vi "FINAL.vi"() -> ()   [LabVIEW 2011]
uses:
  <vilib>/Instr/_visa.llb/VISA Configure Serial Port (Instr).vi
panel:
  out "Light Sensor":dbl(slide) scale=0.0..1500.0
  out "Pressure":dbl(knob) scale=0.0..150000.0
  in  "flow control":u16(ring) items=["None"=0, "XON/XOFF"=1, "RTS/CTS"=2, "DTR/DSR"=4]
  in  "stop bits":u16(ring)=10 items=["1.0"=10, "1.5"=15, "2.0"=20]
  in  "parity":u16(ring) items=["None", "Odd", "Even", "Mark", "Space"]
  in  "data bits":u16=8 min=5 max=8 step=1
  in  "read":bool=TRUE
  out "bytes read":u32
  out "read string":string
  in  "VISA resource name":refnum<visa-resource-name>="COM1"
  in  "baud rate":u32=9600
  out "?":dbl
  out "?":dbl
  out "?":dbl
  out "Temperature  F (SCP1000 sensor)":dbl(slide) scale=0.0..200000.0
  out "?":dbl
  out "Temperature C":dbl(slide) scale=0.0..100.0
  out "Humidity":dbl
  out "?":dbl
  out "?":dbl(knob) scale=0.0..100.0
  out "Temperature  F (SHT15 sensor)":dbl(slide) scale=0.0..100.0
  out "output array":string[](array[string])
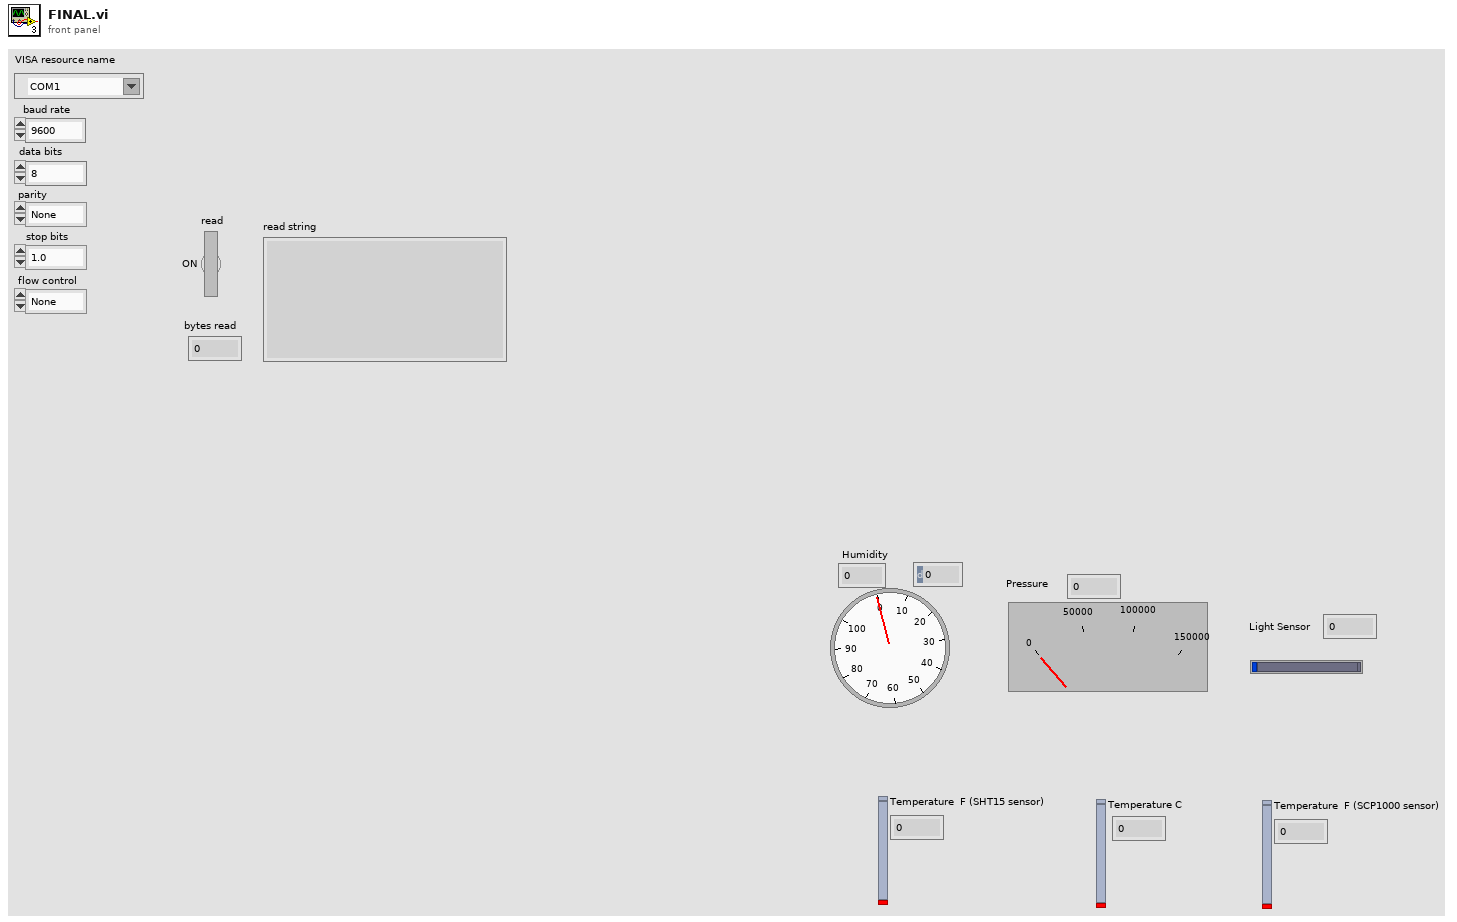
[diagram p1: front panel]
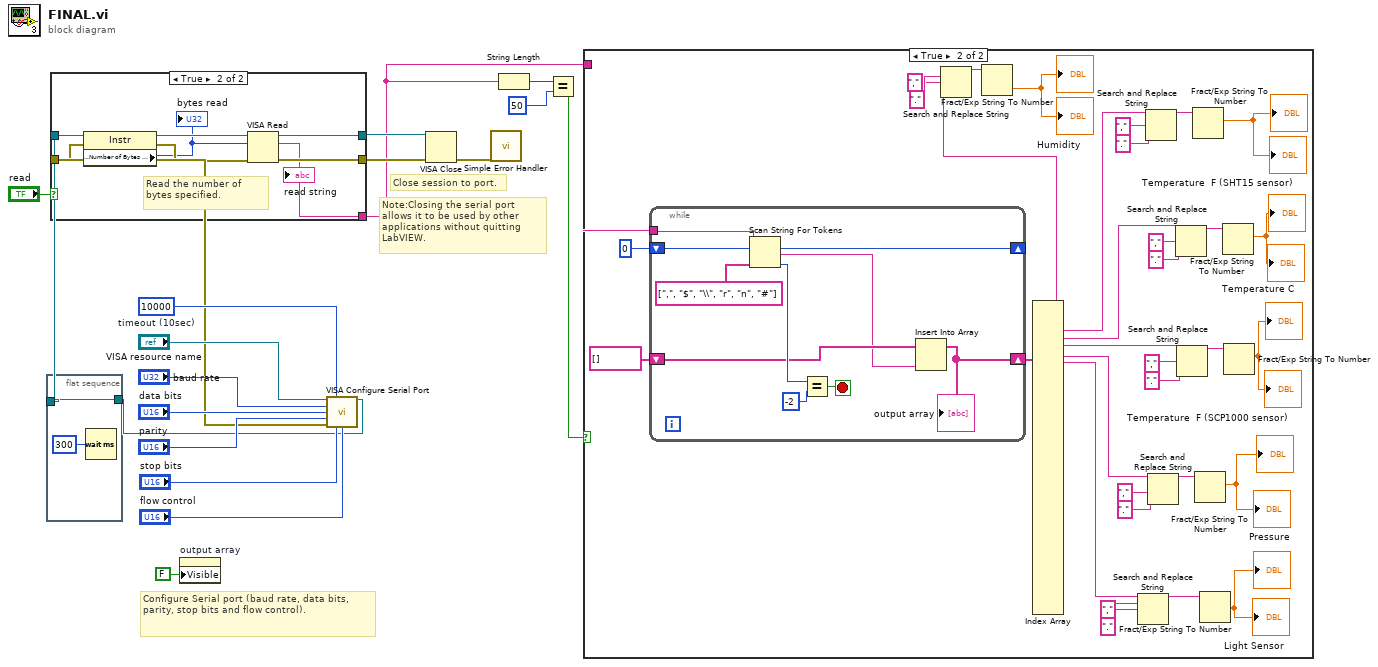
[diagram p0: block diagram]
diagram:
  w12 = u32 10000  # timeout (10sec)
  # "Note:Closing the serial port allows it to be used by other applications without quitting LabVIEW."
  # "Configure Serial port (baud rate, data bits, parity, stop bits and flow control)."
  # "Close session to port."
  n1 = flat-sequence {
    tunnel: [w21] -> w2
    tunnel: w1 -> [w21]
    frame #0 {
      n2 = Wait (ms)(milliseconds to wait=u32 300) -> ()  [unwired: 1 out]
    }
  }
  n3 = property on="output array" class="Arr (strict)"("Visible"=FALSE) -> ()  [unwired: 2 in, 2 out]
  n4 = call-poly "VISA Configure Serial Port"("VISA resource name"="VISA resource name", "timeout (10sec)"=w12, "baud rate (9600)"="baud rate", "data bits (8)"="data bits", "parity (0:none)"="parity", "stop bits (10: 1 bit)"="stop bits", "flow control (0:none)"="flow control") -> ("VISA resource name out"=w1:refnum<visa-resource-name>, "error out"=w3:errorcluster)  [unwired: 2 in, 5 out]
  n5 = case shown="True" "read" {
    tunnel: w3 -> [w23 w27]
    tunnel: [w23 w31] -> w16
    tunnel: [w22 w30] -> w15
    tunnel: w2 -> [w22 w29]
    tunnel: [_ w24] -> w5
    frame False {
    }
    frame True {
      # "Read the number of bytes specified."
      n6 = property class="Instr"(reference=w29, error in=w27) -> (reference out=w28:refnum<visa-resource-name>, error out=w26:errorcluster, "Serial Settings:Number of Bytes at Serial Port"=w25:u32)
      "bytes read" <- w25
      n7 = VISA Read(VISA resource name=w28, byte count=w25, error in (no error)=w26) -> (VISA resource name out=w30:refnum<visa-resource-name>, read buffer=w24:string, error out=w31:errorcluster)  [unwired: 1 out]
      "read string" <- w24
    }
  }
  n8 = VISA Close(VISA resource name=w15, error in (no error)=w16) -> (error out=w14:errorcluster)
  n9 = call <vilib>:"Simple Error Handler.vi"("error in (no error)"=w14) -> ()  [unwired: 1 in, 8 out]
  n10 = String Length(string=w5) -> (length=w8:i32)
  n11 = Equal?(x=w8, y=50) -> (x = y?=w6:bool)
  n12 = case shown="True" w6 {
    tunnel: w5 -> [_ w39]
    frame False {
    }
    frame True {
      n13 = while {
        shift-right: [w68] -> w62
        shift-left: string[] [] -> [w66]
        shift-right: [w69] -> _
        shift-left: 0 -> [w74]
        tunnel: w39 -> [w67]
        stop <- w70 stop-if-true
        n14 = Scan String For Tokens(6:string[] [",", "$", "\\", "r", "n", "#"], 8:w74, 9:w67) -> (0:w72:i32, 1:w65:string, 2:w69:i32)  [unwired: 3 in, 1 out]
        n15 = Equal?(x=w72, y=-2) -> (x = y?=w70:bool)
        n16 = Insert Into Array(array=w66, new element=w65) -> (w68:string[])  [unwired: 1 in]
        "output array" <- w68
      }
      n17 = Index Array(array=w62) -> (element #1=w56:string, element #2=w60:string, element #3=w45:string, element #5=w38:string, element #6=w36:string)  [unwired: 37 in, 32 out]
      n18 = Search and Replace String(input string=w56, search string=".", replace string="," ("replace string (\"\")")) -> (result string=w58:string)  [unwired: 5 in, 3 out]
      n19 = Fract/Exp String To Number(string=w58) -> (number=→"?" →"Humidity":dbl)  [unwired: 3 in, 1 out]
      n20 = Search and Replace String(input string=w36, search string=".", replace string="," ("replace string (\"\")")) -> (result string=w41:string)  [unwired: 5 in, 3 out]
      n21 = Search and Replace String(input string=w60, search string=".", replace string="," ("replace string (\"\")")) -> (result string=w61:string)  [unwired: 5 in, 3 out]
      n22 = Search and Replace String(input string=w38, search string=".", replace string="," ("replace string (\"\")")) -> (result string=w44:string)  [unwired: 5 in, 3 out]
      n23 = Search and Replace String(input string=w45, search string=".", replace string="," ("replace string (\"\")")) -> (result string=w53:string)  [unwired: 5 in, 3 out]
      n24 = Search and Replace String(input string=w38, search string=".", replace string="," ("replace string (\"\")")) -> (result string=w49:string)  [unwired: 5 in, 3 out]
      n25 = Fract/Exp String To Number(string=w61) -> (number=→"Temperature  F (SHT15 sensor)" →"?":dbl)  [unwired: 3 in, 1 out]
      n26 = Fract/Exp String To Number(string=w44) -> (number=→"?" →"Pressure":dbl)  [unwired: 3 in, 1 out]
      n27 = Fract/Exp String To Number(string=w41) -> (number=→"?" →"Light Sensor":dbl)  [unwired: 3 in, 1 out]
      n28 = Fract/Exp String To Number(string=w53) -> (number=→"Temperature C" →"?":dbl)  [unwired: 3 in, 1 out]
      n29 = Fract/Exp String To Number(string=w49) -> (number=→"Temperature  F (SCP1000 sensor)" →"?":dbl)  [unwired: 3 in, 1 out]
    }
  }
